vi "append.vi"(8 "error in (no error)":errorcluster, 10 "data":dbl, 11 "node in":refnum<class "node.lvclass">) -> (0 "error out":errorcluster, 3 "node out":refnum<class "node.lvclass">)   [LabVIEW 2014, in "Linked List.lvlib" / "node.lvclass"]
uses:
  node.lvclass
  node.lvclass/node.ctl
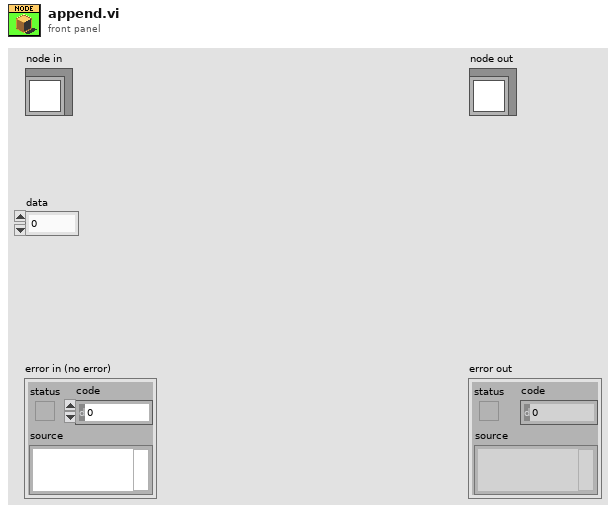
[diagram p1: front panel]
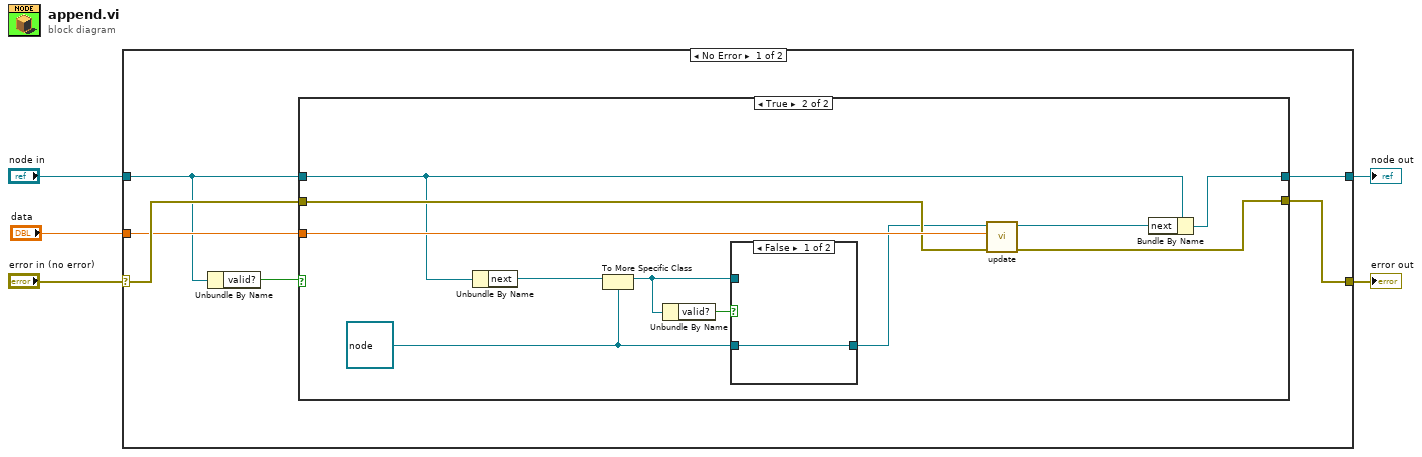
[diagram p0: block diagram]
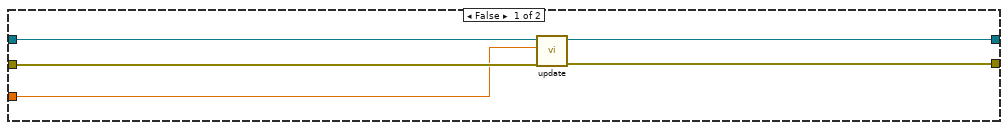
[diagram p2: hidden frame]
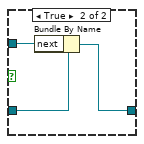
[diagram p3: hidden frame]
diagram:
  n1 = case shown="No Error" "error in (no error)" {
    selector: "error in (no error)" -> [w11 w33]
    tunnel: [w9 w33] -> w4
    tunnel: [w10 w32] -> w2
    tunnel: "node in" -> [w7 w32]
    tunnel: "data" -> [w8 _]
    frame No Error {
      n2 = Unbundle By Name(w7) -> ("valid?"=w6:bool)
      n3 = case shown="True" w6 {
        tunnel: w7 -> [w16 w22]
        tunnel: [w12 w18] -> w10
        tunnel: w11 -> [w15 w26]
        tunnel: [w14 w25] -> w9
        tunnel: w8 -> [w13 w27]
        frame False {
          n4 = call-dynamic "update.vi"("error in (no error)"=w15, "data"=w13, "node in"=w16) -> ("error out"=w14:errorcluster, "node out"=w12:refnum<class "node.lvclass">)  [unwired: 7 in]
        }
        frame True {
          w24 = refnum<class "node.lvclass"> refnum ("Linked List.lvlib:node")
          n5 = Unbundle By Name(w22) -> ("next"=w21:refnum<class "base.lvclass">)
          n6 = To More Specific Class(target class=w24, reference=w21) -> (specific class reference=w20:refnum<class "node.lvclass">)  [unwired: 1 in, 1 out]
          n7 = Unbundle By Name(w20) -> ("valid?"=w19:bool)
          n8 = case shown="False" w19 {
            tunnel: w24 -> [w28 w31]
            tunnel: [w28 w30] -> w23
            tunnel: w20 -> [_ w29]
            frame False {
            }
            frame True {
              n9 = Bundle By Name(cluster=w31, "next"=w29) -> (w30:refnum<class "node.lvclass">)
            }
          }
          n10 = call-dynamic "update.vi"("error in (no error)"=w26, "data"=w27, "node in"=w23) -> ("error out"=w25:errorcluster, "node out"=w17:refnum<class "node.lvclass">)  [unwired: 7 in]
          n11 = Bundle By Name(cluster=w22, "next"=w17) -> (w18:refnum<class "node.lvclass">)
        }
      }
    }
    frame Error {
    }
  }
  "error out" <- w4
  "node out" <- w2
